vi "queue_state_&_argument (Array).vi"(6 "Priority? Array":bool[](array[boolean]), 8 "error in (no error)":errorcluster, 10 "state:argument array":string[](array[string]), 11 "Queue in":refnum<queue>) -> (0 "error out":errorcluster, 3 "Queue out":refnum<queue>)   [LabVIEW 2024]
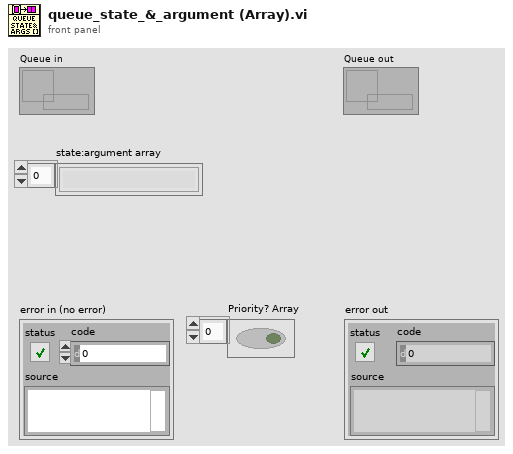
[diagram p1: front panel]
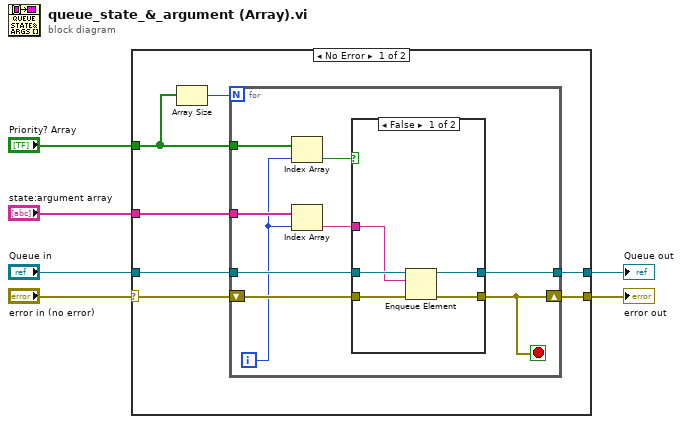
[diagram p0: block diagram]
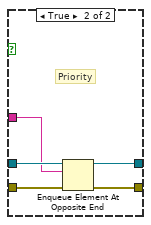
[diagram p2: hidden frame]
diagram:
  n1 = case shown="No Error" "error in (no error)" {
    selector: "error in (no error)" -> [w13 w34]
    tunnel: [w12 w34] -> w4
    tunnel: "Queue in" -> [w11 w33]
    tunnel: [w10 w33] -> w6
    tunnel: "Priority? Array" -> [w7 _]
    tunnel: "state:argument array" -> [w9 _]
    frame No Error {
      n2 = Array Size(array=w7) -> (size(s)=w8:i32)
      n3 = for {
        N: w8 -> [_]
        shift-right: [w19] -> w12
        shift-left: w13 -> [w22]
        tunnel: w11 -> [w21]
        tunnel: [w20] -> w10
        tunnel: w9 -> [w16]
        tunnel: w7 -> [w18]
        i -> [w14]
        stop <- w19 stop-if-true
        n4 = Index Array(array=w18, index=w14) -> (element=w17:bool)
        n5 = Index Array(array=w16, index=w14) -> (element=w15:string)
        n6 = case shown="False" w17 {
          tunnel: w22 -> [w27 w32]
          tunnel: w21 -> [w26 w30]
          tunnel: [w25 w29] -> w20
          tunnel: w15 -> [w24 w28]
          tunnel: [w23 w31] -> w19
          frame False {
            n7 = Enqueue Element(queue=w26, element=w24, error in (no error)=w27) -> (queue out=w25:refnum<queue>, error out=w23:errorcluster)  [unwired: 1 in, 1 out]
          }
          frame True {
            # "Priority"
            n8 = Enqueue Element At Opposite End(queue=w30, element=w28, error in (no error)=w32) -> (queue out=w29:refnum<queue>, error out=w31:errorcluster)  [unwired: 1 in, 1 out]
          }
        }
      }
    }
    frame Error {
    }
  }
  "error out" <- w4
  "Queue out" <- w6
